vi "Oscilloscope.vi"() -> ()   [LabVIEW 2021]
uses:
  <userlib>/SciSDK/SciSDK_Labview.lvlib
panel:
  out "Oscilloscope Buffer Out":T1
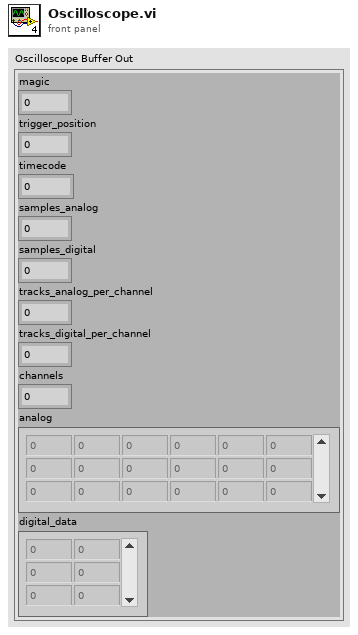
[diagram p1: front panel]
types:
  T1 = cluster{"magic":u32, "trigger_position":u64, "timecode":u64, "samples_analog":u32, "samples_digital":u32, "tracks_analog_per_channel":u32, "tracks_digital_per_channel":u32, "channels":u32, "analog":i32[][], "digital_data":i32[][]}
  T2 = cluster{"Name":string, "Board Model":string, "Handle":u64}
  T3 = cluster{"Oscilloscope Path":string, "Oscilloscope Name":string}
  T4 = cluster{"Board Name":string, "Board Model":string, "Handle":u64}
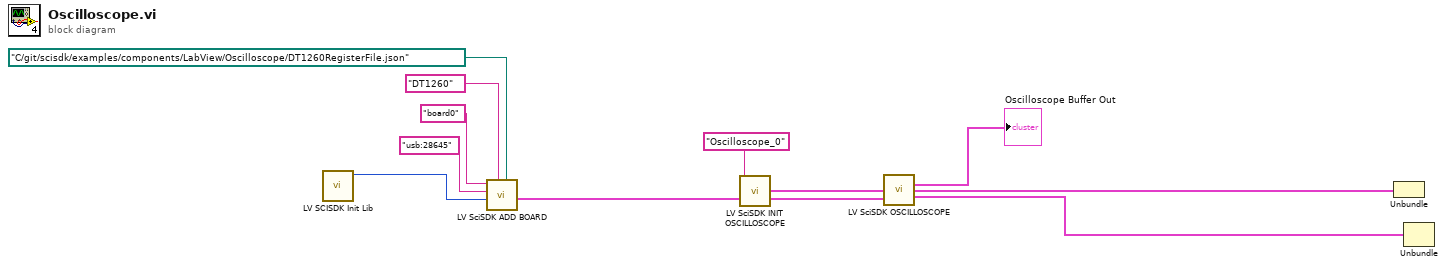
[diagram p0: block diagram]
diagram:
  n1 = call <userlib>:"LV SCISDK Init Lib.vi"() -> ("function return"=w12:u64)  [unwired: 11 in]
  n2 = call <userlib>:"LV SciSDK ADD BOARD.vi"("JsonFile"=path "C:/git/scisdk/examples/components/LabView/Oscilloscope/DT1260RegisterFile.json", "Board Model"="DT1260", "SciSDK Handle"=w12, "DevicePath"="usb:28645", "Name"="board0") -> ("Board Handle Out"=w11:T2)  [unwired: 4 in, 2 out]
  n3 = call <userlib>:"LV SciSDK INIT OSCILLOSCOPE.vi"("Oscilloscope Name"="Oscilloscope_0", "Handle In"=w11) -> ("Oscilloscope Handle Out"=w10:T3, "Board Handle Out"=w9:T4)  [unwired: 15 in, 1 out]
  n4 = call <userlib>:"LV SciSDK OSCILLOSCOPE.vi"("Oscilloscope Handle In"=w10, "Board Handle In"=w9) -> ("Oscilloscope Buffer Out"=→"Oscilloscope Buffer Out":T1, "Oscilloscope Handle Out"=w2:T3, "Board Handle Out"=w1:T4)  [unwired: 9 in, 2 out]
  n5 = Unbundle(w2) -> ()  [unwired: 2 out]
  n6 = Unbundle(w1) -> ()  [unwired: 3 out]
